vi "Increment Survey Point.vi"(0 "Current Point":T1 {"Latitude" format="%#_10g"; "Longitude" format="%#_10g"}, 1 "Point Found":bool, 5 "Image Width (m)":dbl, 7 "Overlap Adjustment":dbl, 9 "Bearing":dbl, 11 "Error In":errorcluster) -> (4 "New Point":T1 {"Latitude" format="%#_10g"; "Longitude" format="%#_10g"}, 15 "Error Out":errorcluster)   [LabVIEW 2014]
uses:
  Lat Long Conversion/Controls/PointLatLon.ctl
  Lat Long Conversion/Increment Bearing.vi
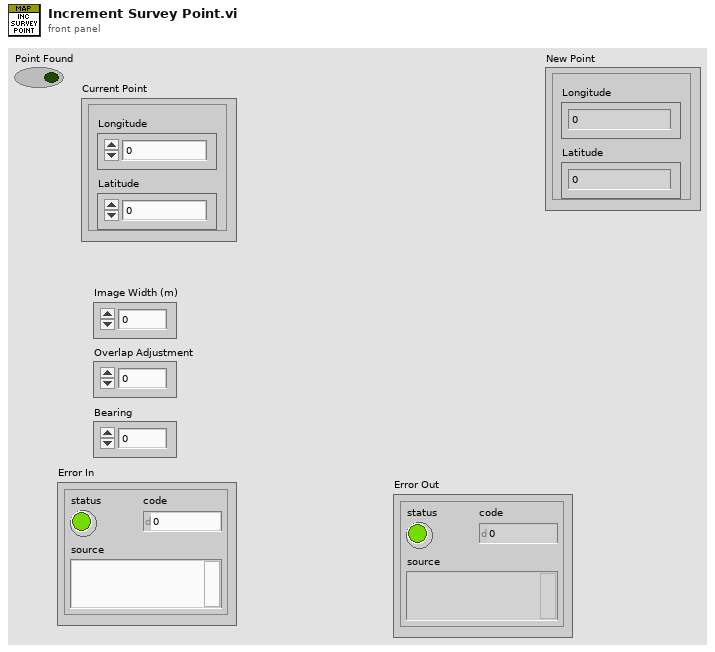
[diagram p1: front panel]
types:
  T1 = typedef "PointLatLon.ctl" = cluster{"Longitude":dbl, "Latitude":dbl}
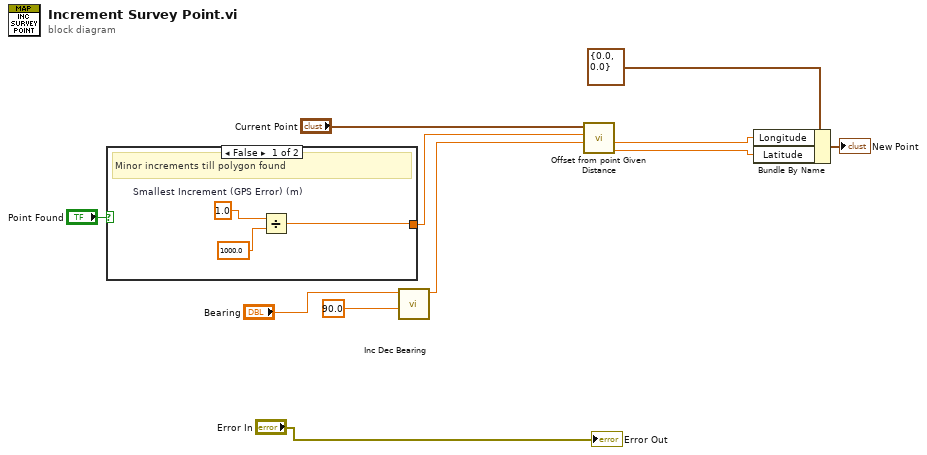
[diagram p0: block diagram]
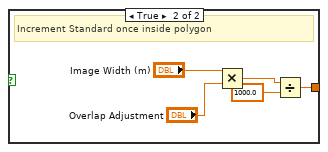
[diagram p2: hidden frame]
diagram:
  n1 = case shown="False" "Point Found" {
    tunnel: [w12 w15] -> w10
    frame False {
      w14 = 1.0  # Smallest Increment (GPS Error) (m)
      # "Minor increments till polygon found"
      n2 = Divide(x=w14, y=1000.0) -> (x/y=w12:dbl)
    }
    frame True {
      # "Increment Standard once inside polygon"
      n3 = Multiply(x="Image Width (m)", y="Overlap Adjustment") -> (x*y=w17:dbl)
      n4 = Divide(x=w17, y=1000.0) -> (x/y=w15:dbl)
    }
  }
  n5 = call-poly "Inc Dec Bearing.vi"("Increment Value"=90.0, "Bearing"="Bearing") -> ("New Bearing"=w7:dbl)  [unwired: 8 in, 1 out]
  n6 = call "Offset from point Given Distance.vi"("Bearing (clockwise from North)"=w7, "Distance (km)"=w10, "Origin Point"="Current Point") -> ("Lat of new point"=w4:dbl, "Lon of new point"=w5:dbl)  [unwired: 5 in, 2 out]
  n7 = Bundle By Name(cluster=T1 {"Longitude"=0.0, "Latitude"=0.0} ("Current Point"), "Longitude"=w5, "Latitude"=w4) -> (→"New Point":T1)
  "Error Out" <- "Error In"
